vi "getSpadInfo.vi"(7 "io_timeout":u16, 8 "error in":errorcluster, 10 "Slave Address (7-bit)":u8, 11 "I2C Ref In":T1) -> (0 "error out":errorcluster, 1 "type_is_aperture":bool, 2 "count":u8, 3 "I2C Ref Out":T1, 4 "status":bool)   [LabVIEW 2018]
uses:
  <vilib>/myRIO/Instrument Drivers/Onboard IO/I2C/typedefs/I2C Reference.ctl
  <vilib>/myRIO/Common/Instrument Driver Framework/Utilities/typedefs/myRIO Generic Hardware Reference.ctl
  <vilib>/myRIO/Common/Instrument Driver Framework/Utilities/typedefs/Hardware Version Enum.ctl
  <vilib>/myRIO/Common/Instrument Driver Framework/Utilities/typedefs/myRIO v1.0 Reference.ctl
  <vilib>/myRIO/Common/Instrument Driver Framework/Utilities/typedefs/Generic FPGA Reference.ctl
  <vilib>/myRIO/Common/Instrument Driver Framework/myRIO v1.0/I2C/typedefs/I2C Channels Enum.ctl
  <vilib>/myRIO/Instrument Drivers/Onboard IO/I2C/typedefs/I2C Configuration.ctl
  <vilib>/myRIO/Instrument Drivers/Onboard IO/I2C/typedefs/I2C Transfer Rate.ctl
  <vilib>/Utility/error.llb/Error Cluster From Error Code.vi
  <vilib>/myRIO/Common/Instrument Driver Framework/myRIO v1.0/I2C/vis/myRIO v1.0 Write I2C.vi
  <vilib>/myRIO/Common/Instrument Driver Framework/myRIO v1.0/I2C/vis/myRIO v1.0 Read I2C.vi
  <vilib>/myRIO/Instrument Drivers/Onboard IO/I2C/I2C.lvlib
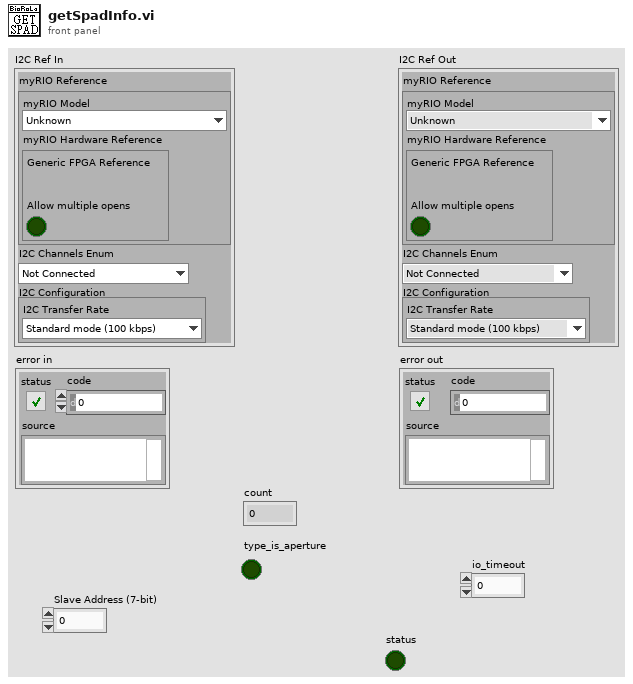
[diagram p1: front panel]
types:
  T1 = typedef "I2C.lvlib/I2C Reference.ctl" = cluster{"myRIO Reference":T2, "I2C Channels Enum":T6, "I2C Configuration":T7}
  T2 = typedef "myRIO Generic Hardware Reference.ctl" = cluster{"myRIO Model":T3, "myRIO Hardware Reference":T4}
  T3 = typedef "Hardware Version Enum.ctl" = enum16{"Unknown", "myRIO-1900", "myRIO-1950", "roboRIO", "NI ELVIS RIO CM", "ELVIS III"}
  T4 = typedef "myRIO v1.0 Reference.ctl" = cluster{"Generic FPGA Reference":T5, "Allow multiple opens":bool}
  T5 = typedef "Generic FPGA Reference.ctl" = refnum<k20>
  T6 = typedef "I2C Channels Enum.ctl" = enum16{"Not Connected", "A/I2C", "B/I2C", "I2C/I2C"}
  T7 = typedef "I2C.lvlib/I2C Configuration.ctl" = cluster{"I2C Transfer Rate":T8}
  T8 = typedef "I2C.lvlib/I2C Transfer Rate.ctl" = enum16{"Standard mode (100 kbps)", "Fast mode (400 kbps)"}
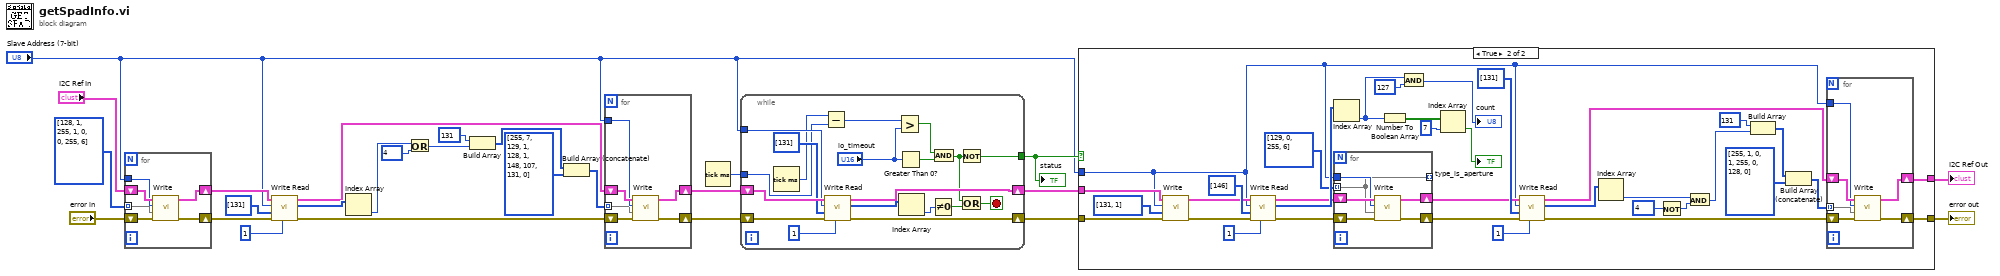
[diagram p0: block diagram]
diagram:
  n1 = for {
    shift-right: [w29] -> w4
    shift-left: "error in" -> [w31]
    shift-right: [w30] -> w3
    shift-left: "I2C Ref In" -> [w32]
    tunnel: u8[][] [[128, 1], [255, 1], [0, 0], [255, 6]] -> [w28] mode=indexing
    tunnel: "Slave Address (7-bit)" -> [w27]
    n2 = call <vilib>:"Write.vi"("error in (no error)"=w31, "Bytes to Write"=w28, "Slave Address (7-bit)"=w27, "I2C Ref In"=w32) -> ("error out"=w29:errorcluster, "I2C Ref Out"=w30:T1)  [unwired: 6 in]
  }
  n3 = call <vilib>:"Write Read.vi"("Byte Count"=u32 1, "error in (no error)"=w4, "Bytes to Write"=u8[] [131], "Slave Address (7-bit)"="Slave Address (7-bit)", "I2C Ref In"=w3) -> ("error out"=w16:errorcluster, "Bytes Read"=w24:u8[], "I2C Ref Out"=w17:T1)  [unwired: 3 in]
  n4 = Index Array(array=w24) -> (element=w23:u8)  [unwired: 1 in]
  n5 = Or(x=w23, y=u8 4) -> (x .or. y?=w21:u8)
  n6 = Build Array(u8 131, w21) -> (w19:u8[])
  n7 = Build Array (concatenate)(w19, u8[][] [[255, 7], [129, 1], [128, 1], [148, 107], [131, 0]]) -> (w15:u8[][])
  n8 = for {
    shift-right: [w33] -> w12
    shift-left: w16 -> [w37]
    shift-right: [w34] -> w13
    shift-left: w17 -> [w38]
    tunnel: "Slave Address (7-bit)" -> [w36]
    tunnel: w15 -> [w35] mode=indexing
    n9 = call <vilib>:"Write.vi"("error in (no error)"=w37, "Bytes to Write"=w35, "Slave Address (7-bit)"=w36, "I2C Ref In"=w38) -> ("error out"=w33:errorcluster, "I2C Ref Out"=w34:T1)  [unwired: 6 in]
  }
  n10 = Tick Count (ms)() -> (millisecond timer value=w14:u32)
  n11 = while {
    tunnel: w14 -> [w48]
    shift-right: [w54] -> w11
    shift-left: w13 -> [w57]
    shift-right: [w53] -> w10
    shift-left: w12 -> [w56]
    tunnel: "Slave Address (7-bit)" -> [w55]
    tunnel: [w39] -> w7
    stop <- w42 stop-if-true
    n12 = Tick Count (ms)() -> (millisecond timer value=w47:u32)
    n13 = Subtract(x=w47, y=w48) -> (x-y=w46:u32)
    n14 = call <vilib>:"Write Read.vi"("Byte Count"=u32 1, "error in (no error)"=w56, "Bytes to Write"=u8[] [131], "Slave Address (7-bit)"=w55, "I2C Ref In"=w57) -> ("error out"=w53:errorcluster, "Bytes Read"=w49:u8[], "I2C Ref Out"=w54:T1)  [unwired: 3 in]
    n15 = Greater?(x=w46, y="io_timeout") -> (0:w45:bool)
    n16 = Greater Than 0?(x="io_timeout") -> (x > 0?=w43:bool)
    n17 = Index Array(array=w49) -> (element=w50:u8)  [unwired: 1 in]
    n18 = Not Equal To 0?(x=w50) -> (x != 0?=w41:bool)
    n19 = And(x=w45, y=w43) -> (x .and. y?=w40:bool)
    n20 = Not(x=w40) -> (.not. x?=w39:bool)
    n21 = Or(x=w40, y=w41) -> (x .or. y?=w42:bool)
  }
  "status" <- w7
  n22 = case shown="True" w7 {
    tunnel: w11 -> [w59 w94]
    tunnel: w10 -> [w58 w93]
    tunnel: "Slave Address (7-bit)" -> [_ w60]
    tunnel: [w59 w67] -> w9
    tunnel: [w58 w66] -> w8
    frame False {
    }
    frame True {
      n23 = call <vilib>:"Write.vi"("error in (no error)"=w93, "Bytes to Write"=u8[] [131, 1], "Slave Address (7-bit)"=w60, "I2C Ref In"=w94) -> ("error out"=w88:errorcluster, "I2C Ref Out"=w89:T1)  [unwired: 6 in]
      n24 = call <vilib>:"Write Read.vi"("Byte Count"=u32 1, "error in (no error)"=w88, "Bytes to Write"=u8[] [146], "Slave Address (7-bit)"=w60, "I2C Ref In"=w89) -> ("error out"=w64:errorcluster, "Bytes Read"=w87:u8[], "I2C Ref Out"=w65:T1)  [unwired: 3 in]
      n25 = Index Array(array=w87) -> (element=w84:u8)  [unwired: 1 in]
      n26 = for {
        shift-right: [w96] -> w63
        shift-left: w64 -> [w99]
        shift-right: [w97] -> w62
        shift-left: w65 -> [w100]
        tunnel: w60 -> [w98]
        tunnel: [w95] -> _ mode=indexing
        tunnel: u8[][] [[129, 0], [255, 6]] -> [w95] mode=indexing
        n27 = call <vilib>:"Write.vi"("error in (no error)"=w99, "Bytes to Write"=w95, "Slave Address (7-bit)"=w98, "I2C Ref In"=w100) -> ("error out"=w96:errorcluster, "I2C Ref Out"=w97:T1)  [unwired: 6 in]
      }
      n28 = Number To Boolean Array(number=w84) -> (Boolean array=w83:bool[])
      n29 = And(x=w84, y=u8 127) -> (x .and. y?=→"count":u8)
      n30 = Index Array(array=w83, index=7) -> (element=→"type_is_aperture":bool)
      n31 = call <vilib>:"Write Read.vi"("Byte Count"=u32 1, "error in (no error)"=w63, "Bytes to Write"=u8[] [131], "Slave Address (7-bit)"=w60, "I2C Ref In"=w62) -> ("error out"=w77:errorcluster, "Bytes Read"=w76:u8[], "I2C Ref Out"=w78:T1)  [unwired: 3 in]
      n32 = Index Array(array=w76) -> (element=w72:u8)  [unwired: 1 in]
      n33 = Not(x=u8 4) -> (.not. x?=w73:u8)
      n34 = And(x=w72, y=w73) -> (x .and. y?=w71:u8)
      n35 = Build Array(u8 131, w71) -> (w70:u8[])
      n36 = Build Array (concatenate)(w70, u8[][] [[255, 1], [0, 1], [255, 0], [128, 0]]) -> (w68:u8[][])
      n37 = for {
        shift-right: [w101] -> w66
        shift-left: w77 -> [w105]
        shift-right: [w102] -> w67
        shift-left: w78 -> [w106]
        tunnel: w60 -> [w104]
        tunnel: w68 -> [w103] mode=indexing
        n38 = call <vilib>:"Write.vi"("error in (no error)"=w105, "Bytes to Write"=w103, "Slave Address (7-bit)"=w104, "I2C Ref In"=w106) -> ("error out"=w101:errorcluster, "I2C Ref Out"=w102:T1)  [unwired: 6 in]
      }
    }
  }
  "I2C Ref Out" <- w9
  "error out" <- w8
